vi "Close Lidar Labview.vi"(8 "error in (no error)":errorcluster) -> (0 "error out":errorcluster)   [LabVIEW 2016]
uses:
  Variables/Labview lidar globals.vi
  <instrlib>/Hokuyo URG Series/Hokuyo URG Series.lvlib
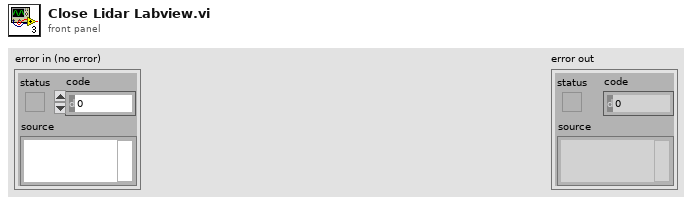
[diagram p1: front panel]
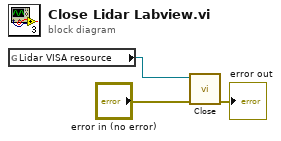
[diagram p0: block diagram]
diagram:
  n1 = global read "Labview lidar globals.vi" "Lidar VISA resource"() -> (w3:refnum<visa-resource-name>)
  n2 = call <instrlib>:"Close.vi"("error in (no error)"="error in (no error)", "VISA resource name"=w3) -> ("error out"=→"error out":errorcluster)  [unwired: 9 in]
